vi "ReadConnected.vi"(8 "error in (no error)":errorcluster, 11 "object in":refnum<class "JuPyter_Client.lvclass">) -> (0 "error out":errorcluster, 2 "Connected?":bool, 3 "object out":refnum<class "JuPyter_Client.lvclass">)   [LabVIEW 2018, in "JuPyter_Client.lvclass"]
uses:
  JuPyter_Client.lvclass
  JuPyter_Client.lvclass/JuPyter_Client.ctl
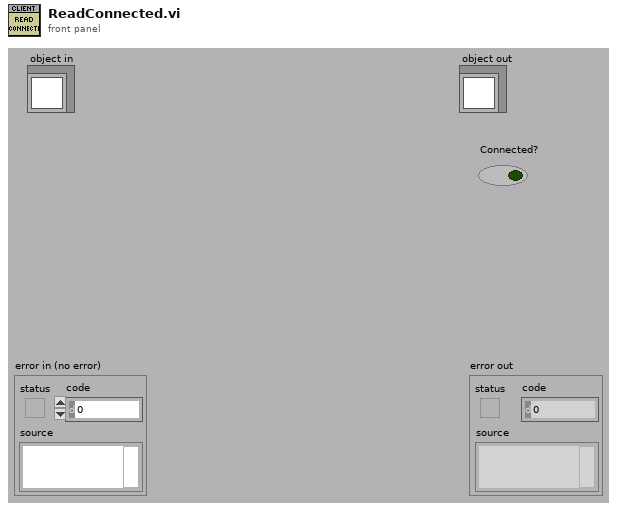
[diagram p1: front panel]
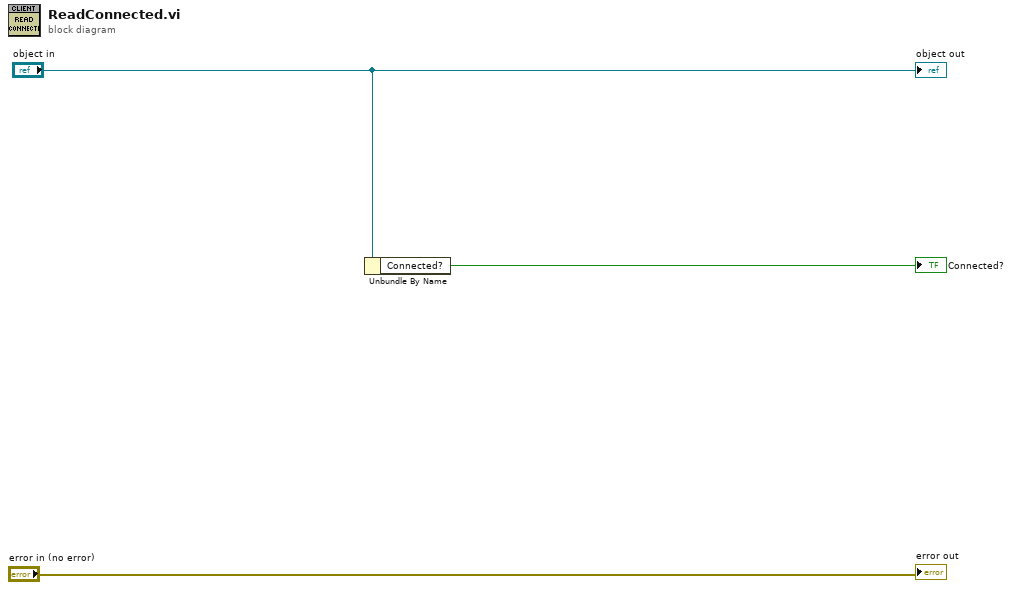
[diagram p0: block diagram]
diagram:
  n1 = Unbundle By Name("object in") -> ("Connected?"=→"Connected?":bool)
  "error out" <- "error in (no error)"
  "object out" <- "object in"
